vi "dronepos.vi"(7 "LabVIEW Web Service Request":refnum<class "Web Request.lvclass">) -> (1 "altitude":dbl, 2 "lon":dbl, 3 "lat":dbl)   [LabVIEW 2014]
uses:
  <vilib>/wsapi/Web Request.lvclass
  DronePi Global Variables.vi
panel:
  # "Use the Web Service Request input terminal to call the VIs on the Web Services palette. Do not remove it from the connector pane unless you don't need access to the palette."
  # "Each additional control wired to the connector pane will be available as an input in the URL. To include an indicator in terminal-mode output (the default setting), it must also be wired to the connector pane."
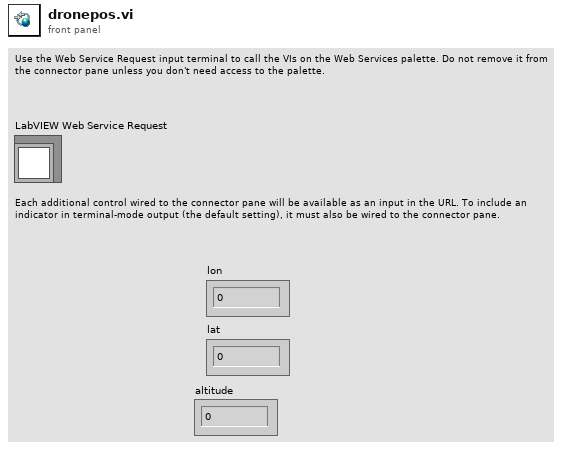
[diagram p1: front panel]
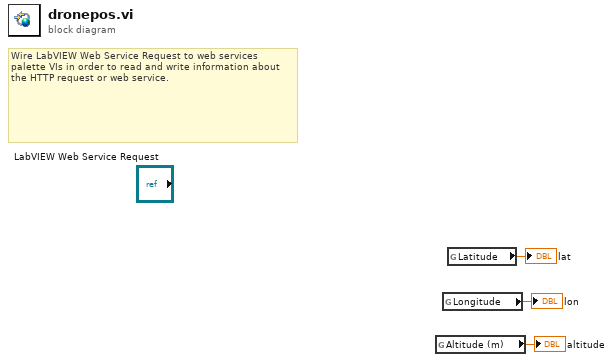
[diagram p0: block diagram]
diagram:
  # "Wire LabVIEW Web Service Request to web services palette VIs in order to read and write information about the HTTP request or web service."
  n1 = global read "DronePi Global Variables.vi" "Altitude (m)"() -> (→"altitude":dbl)
  n2 = global read "DronePi Global Variables.vi" "Longitude"() -> (→"lon":dbl)
  n3 = global read "DronePi Global Variables.vi" "Latitude"() -> (→"lat":dbl)
